vi "ALTS-2015 Write Status Log.vi"(8 "error in (no error)":errorcluster, 11 "Status Input":string) -> (0 "error out":errorcluster)   [LabVIEW 2013]
uses:
  Globals/ALTS-2015 Global Variables.vi
panel:
  out "Message":string
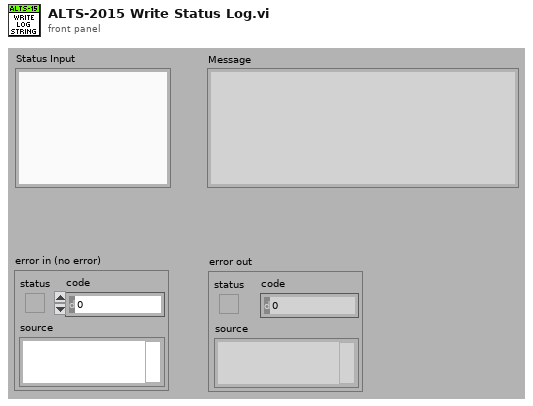
[diagram p1: front panel]
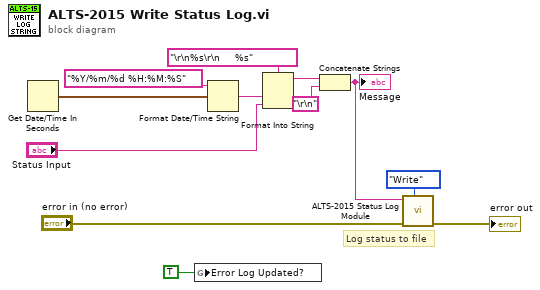
[diagram p0: block diagram]
diagram:
  # "Log status to file"
  n1 = Get Date/Time In Seconds() -> (seconds since 1Jan1904=w8:timestamp)
  n2 = global write "ALTS-2015 Global Variables.vi" "Error Log Updated?"(TRUE ("Exit Troubleshooter VI")) -> ()
  n3 = Format Date/Time String(time format string (%c)="%Y/%m/%d %H:%M:%S", seconds (now)=w8) -> (date/time string=w9:string)  [unwired: 1 out]
  n4 = Format Into String(format string="\r\n%s\r\n     %s", w9, "Status Input") -> (resulting string=w11:string)  [unwired: 2 in, 1 out]
  n5 = Concatenate Strings(w11, "\r\n") -> (w4:string)
  "Message" <- w4
  n6 = call "ALTS-2015 Status Log Module.vi"("Options"=enum16{"Init", "Write", "Close"}."Write", "error in"="error in (no error)", "Text to  Log"=w4) -> ("error out"=→"error out":errorcluster)  [unwired: 8 in]
